vi "Configure Input Parameters.vi"(0 "VISA resource name":refnum<visa-resource-name>, 1 "Input Name (\"\")":string, 2 "Enable Compensation (F: Disable)":bool, 3 "Sensor Excitation (0:1 mV)":u16(ring) items=["1 mV", "10 mV"], 5 "Input (0:A)":u16(ring) items=["A", "B", "C", "D", "D2", "D3", "D4", "D5"], 7 "Sensor Type and Range (0:Disabled)":u16(ring) items=["Disabled", "Diode 2.5 V (Silicon)", "Diode 10 V (GaAlAs)", "PTC RTD Autorange", "PTC RTD 10 Ohm", "PTC RTD 30 Ohm", "PTC RTD 100 Ohm", "PTC RTD 300 Ohm", "PTC RTD 1 kOhm", "PTC RTD 3 kOhm", "PTC RTD 10 kOhm", "NTC RTD Autorange", "NTC RTD 10 Ohm", "NTC RTD 30 Ohm", "NTC RTD 100 Ohm", "NTC RTD 300 Ohm", "NTC RTD 1 kOhm", "NTC RTD 3 kOhm", "NTC RTD 10 kOhm", "NTC RTD 30 kOhm", "NTC RTD 100 kOhm", "NTC RTD 300 kOhm", "Thermocouple", "Capacitor 15nF", "Capacitor 150nF"], 9 "Diode Current (0:10 uA)":u16(ring) items=["10 uA", "1 mA"], 11 "error in (no error)":errorcluster, 12 "Preferred Units (1:Kelvin)":u16(ring)=1 items=["Kelvin"=1, "Celsius"=2, "Sensor Units"=3], 13 "Curve (0:None)":u16(ring) items=["None"=0, "DT-470"=1, "DT-670"=2, "DT-500-D"=3, "DT-500-E1"=4, "PT-100"=6, "PT-1000"=7, "RX-102A-AA"=8, "RX-202A-AA"=9, "Type K"=12, "Type E"=13, "Type T"=14, "AuFe 0.03%"=15, "AuFe 0.07%"=16, "User 21"=21, "User 22"=22, "User 23"=23, "User 24"=24, "User 25"=25, "User 26"=26, "User 27"=27, "User 28"=28, "User 29"=29, "User 30"=30, "User 31"=31, "User 32"=32, "User 33"=33, "User 34"=34, "User 35"=35, "User 36"=36, "User 37"=37, "User 38"=38, "User 39"=39, "User 40"=40, "User 41"=41, "User 42"=42, "User 43"=43, "User 44"=44, "User 45"=45, "User 46"=46, "User 47"=47, "User 48"=48, "User 49"=49, "User 50"=50, "User 51"=51, "User 52"=52, "User 53"=53, "User 54"=54, "User 55"=55, "User 56"=56, "User 57"=57, "User 58"=58, "User 59"=59], 14 "Temperature Limit (0)":u16) -> (4 "VISA resource name out":refnum<visa-resource-name>, 15 "error out":errorcluster)   [LabVIEW 2010, in "Lake Shore 350.lvlib"]
doc: "Configures the sensor input parameters. The Model 350 supports a variety of temperature sensors sold by Lake Shore and other manufacturers. An appropriate sensor type must be selected for each of the four inputs (eight, if using the 3062 option card). If the exact sensor model is not shown, use the sensor input types chart in section 4 of the 350 User's Manual."
uses:
  <instrlib>/Lake Shore 350/Lake Shore 350.lvlib
  Instance           1 34Saved   Configure Input Parameters .vi
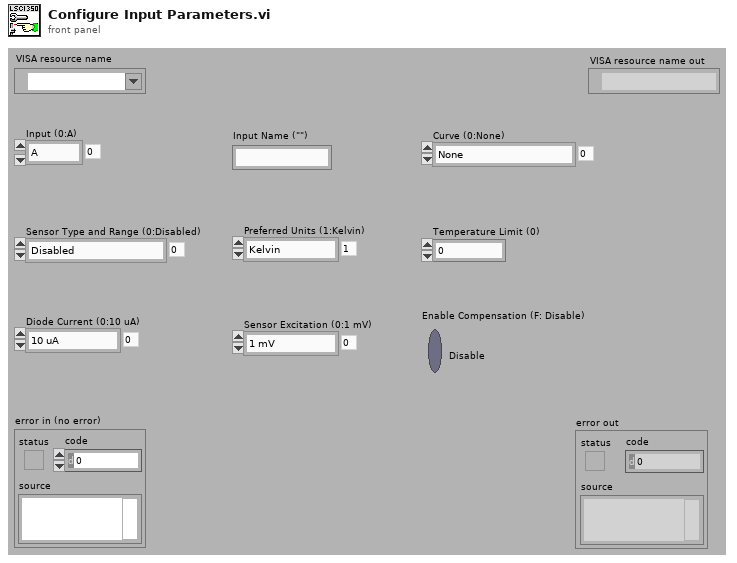
[diagram p1: front panel]
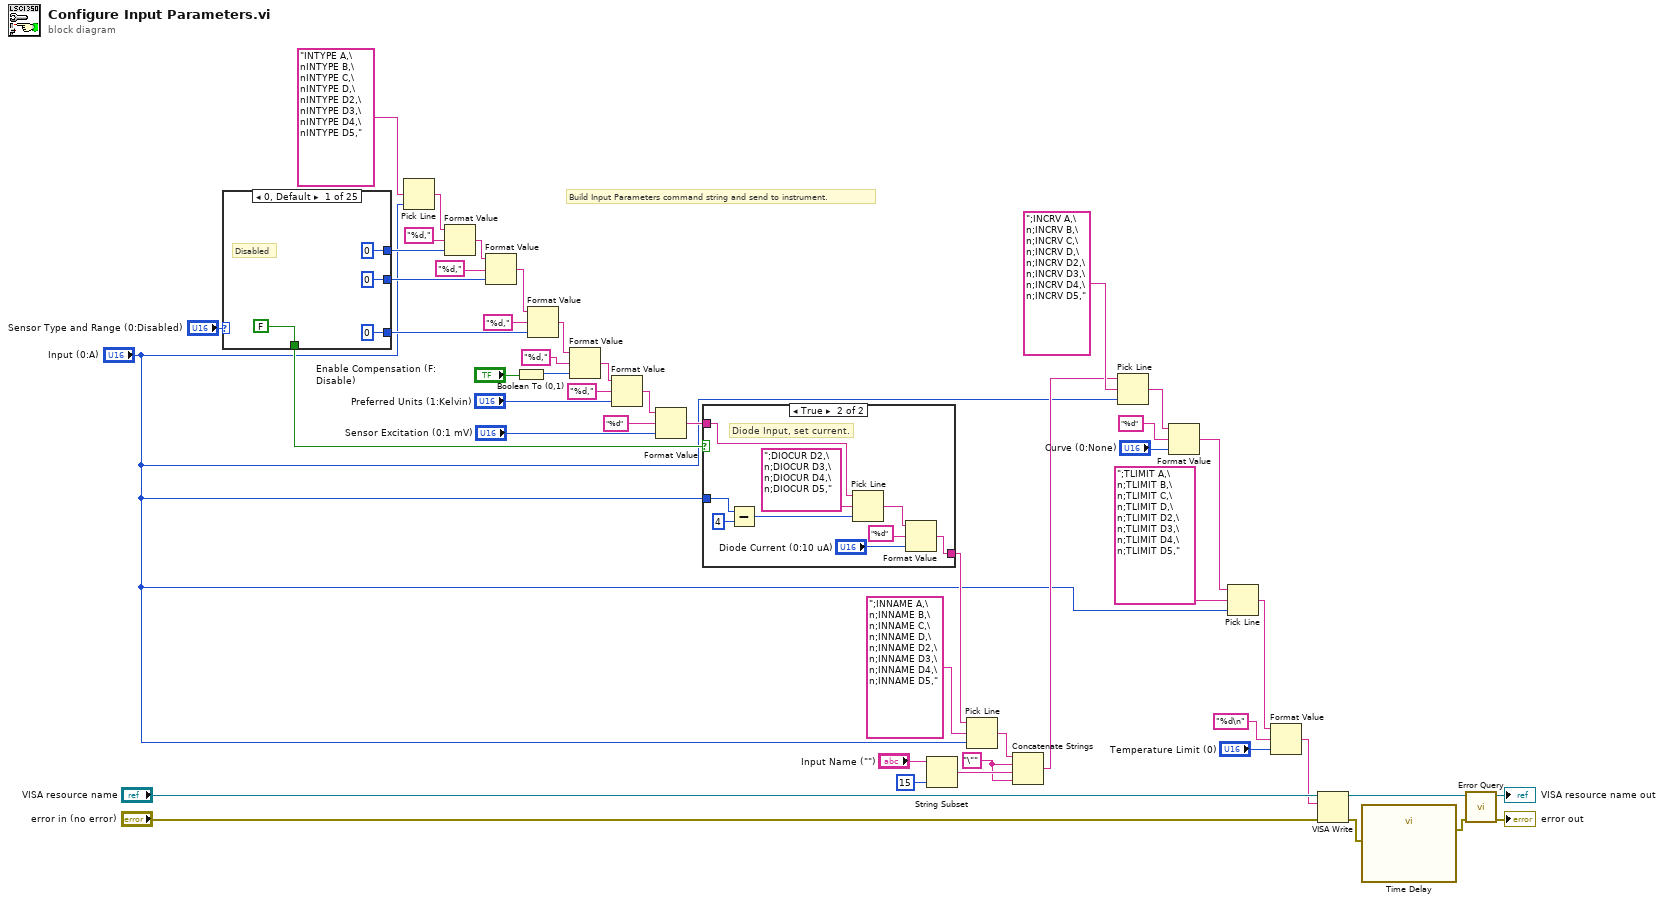
[diagram p0: block diagram]
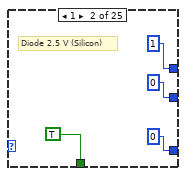
[diagram p3: hidden frame]
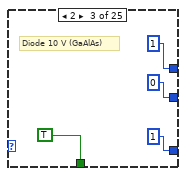
[diagram p4: hidden frame]
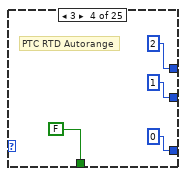
[diagram p5: hidden frame]
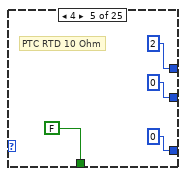
[diagram p6: hidden frame]
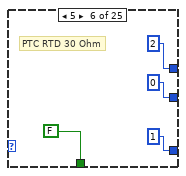
[diagram p7: hidden frame]
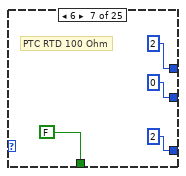
[diagram p8: hidden frame]
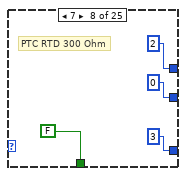
[diagram p9: hidden frame]
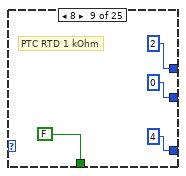
[diagram p10: hidden frame]
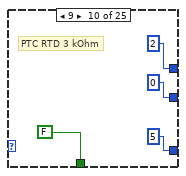
[diagram p11: hidden frame]
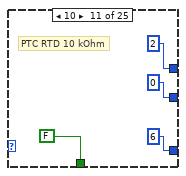
[diagram p12: hidden frame]
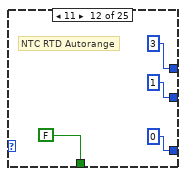
[diagram p13: hidden frame]
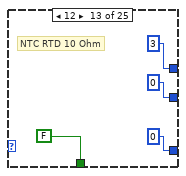
[diagram p14: hidden frame]
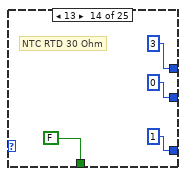
[diagram p15: hidden frame]
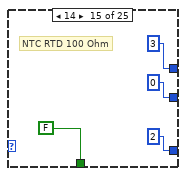
[diagram p16: hidden frame]
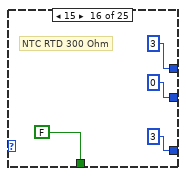
[diagram p17: hidden frame]
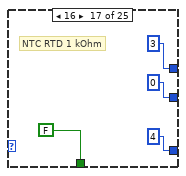
[diagram p18: hidden frame]
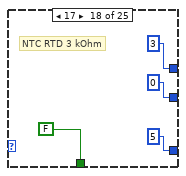
[diagram p19: hidden frame]
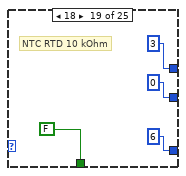
[diagram p20: hidden frame]
diagram:
  w12 = "\""
  # "Build Input Parameters command string and send to instrument."
  n1 = case shown="0, Default" "Sensor Type and Range (0:Disabled)" {
    tunnel: [0 1 1 2 2 2 2 2 2 2 2 3 3 3 3 3 3 3 3 3 3 3 4 5 5] -> w23
    tunnel: [0 0 0 1 0 0 0 0 0 0 0 1 0 0 0 0 0 0 0 0 0 0 0 0 0] -> w22
    tunnel: [0 0 1 0 0 1 2 3 4 5 6 0 0 1 2 3 4 5 6 7 8 9 0 0 1] -> w21
    tunnel: [FALSE TRUE TRUE FALSE FALSE FALSE FALSE FALSE FALSE FALSE FALSE FALSE FALSE FALSE FALSE FALSE FALSE FALSE FALSE FALSE FALSE FALSE FALSE FALSE FALSE] -> w7
    frame 0, Default {
      # "Disabled"
    }
    frame 1 {
      # "Diode 2.5 V (Silicon)"
    }
    frame 2 {
      # "Diode 10 V (GaAlAs)"
    }
    frame 3 {
      # "PTC RTD Autorange"
    }
    frame 4 {
      # "PTC RTD 10 Ohm"
    }
    frame 5 {
      # "PTC RTD 30 Ohm"
    }
    frame 6 {
      # "PTC RTD 100 Ohm"
    }
    frame 7 {
      # "PTC RTD 300 Ohm"
    }
    frame 8 {
      # "PTC RTD 1 kOhm"
    }
    frame 9 {
      # "PTC RTD 3 kOhm"
    }
    frame 10 {
      # "PTC RTD 10 kOhm"
    }
    frame 11 {
      # "NTC RTD Autorange"
    }
    frame 12 {
      # "NTC RTD 10 Ohm"
    }
    frame 13 {
      # "NTC RTD 30 Ohm"
    }
    frame 14 {
      # "NTC RTD 100 Ohm"
    }
    frame 15 {
      # "NTC RTD 300 Ohm"
    }
    frame 16 {
      # "NTC RTD 1 kOhm"
    }
    frame 17 {
      # "NTC RTD 3 kOhm"
    }
    frame 18 {
      # "NTC RTD 10 kOhm"
    }
    frame 19 {
      # "NTC RTD 30 kOhm"
    }
    frame 20 {
      # "NTC RTD 100 kOhm"
    }
    frame 21 {
      # "NTC RTD 300 kOhm"
    }
    frame 22 {
      # "Thermocouple"
    }
    frame 23 {
      # "Capacitor 15nF"
    }
    frame 24 {
      # "Capacitor 150 nF"
    }
  }
  n2 = Pick Line(multi-line string="INTYPE A,\nINTYPE B,\nINTYPE C,\nINTYPE D,\nINTYPE D2,\nINTYPE D3,\nINTYPE D4,\nINTYPE D5,", line index="Input (0:A)") -> (output string=w41:string)  [unwired: 1 in]
  n3 = Format Value(string ("")=w41, format string="%d,", value (0)=w23) -> (output string=w31:string)
  n4 = Format Value(string ("")=w31, format string="%d,", value (0)=w22) -> (output string=w29:string)
  n5 = Boolean To (0,1)(Boolean="Enable Compensation (F: Disable)") -> (0, 1=w38:i16)
  n6 = Format Value(string ("")=w29, format string="%d,", value (0)=w21) -> (output string=w28:string)
  n7 = Format Value(string ("")=w28, format string="%d,", value (0)=w38) -> (output string=w26:string)
  n8 = Format Value(string ("")=w26, format string="%d,", value (0)="Preferred Units (1:Kelvin)") -> (output string=w4:string)
  n9 = Format Value(string ("")=w4, format string="%d", value (0)="Sensor Excitation (0:1 mV)") -> (output string=w6:string)
  n10 = case shown="True" w7 {
    tunnel: [w150 w159] -> w8
    tunnel: w6 -> [w150 w154]
    tunnel: "Input (0:A)" -> [_ w153]
    frame False {
      # "Not Diode Input, do not set current."
    }
    frame True {
      # "Diode Input, set current."
      n11 = Subtract(x=w153, y=u16 4) -> (x-y=w152:u16)
      n12 = Pick Line(string ("")=w154, multi-line string=";DIOCUR D2,\n;DIOCUR D3,\n;DIOCUR D4,\n;DIOCUR D5,", line index=w152) -> (output string=w157:string)
      n13 = Format Value(string ("")=w157, format string="%d", value (0)="Diode Current (0:10 uA)") -> (output string=w159:string)
    }
  }
  n14 = String Subset(string="Input Name (\"\")", length (rest)=15) -> (substring=w13:string)  [unwired: 1 in]
  n15 = Pick Line(string ("")=w8, multi-line string=";INNAME A,\n;INNAME B,\n;INNAME C,\n;INNAME D,\n;INNAME D2,\n;INNAME D3,\n;INNAME D4,\n;INNAME D5,", line index="Input (0:A)") -> (output string=w18:string)
  n16 = Concatenate Strings(w18, w12, w13, w12) -> (w2:string)
  n17 = Pick Line(string ("")=w2, multi-line string=";INCRV A,\n;INCRV B,\n;INCRV C,\n;INCRV D,\n;INCRV D2,\n;INCRV D3,\n;INCRV D4,\n;INCRV D5,", line index="Input (0:A)") -> (output string=w36:string)
  n18 = Format Value(string ("")=w36, format string="%d", value (0)="Curve (0:None)") -> (output string=w9:string)
  n19 = Pick Line(string ("")=w9, multi-line string=";TLIMIT A,\n;TLIMIT B,\n;TLIMIT C,\n;TLIMIT D,\n;TLIMIT D2,\n;TLIMIT D3,\n;TLIMIT D4,\n;TLIMIT D5,", line index="Input (0:A)") -> (output string=w15:string)
  n20 = Format Value(string ("")=w15, format string="%d\n", value (0)="Temperature Limit (0)") -> (output string=w10:string)
  n21 = VISA Write(VISA resource name="VISA resource name", write buffer=w10, error in (no error)="error in (no error)") -> (VISA resource name out=w47:refnum<visa-resource-name>, error out=w34:errorcluster)  [unwired: 1 out]
  n22 = call "Time Delay"("error in (no error)"=w34) -> ("error out"=w33:errorcluster)  [unwired: 10 in]
  n23 = call <instrlib>:"Error Query.vi"("error in (no error)"=w33, "VISA resource name"=w47) -> ("error out"=→"error out":errorcluster, "VISA resource name out"=→"VISA resource name out":refnum<visa-resource-name>)  [unwired: 7 in, 1 out]
